vi "InitializeHardware_RT.vi"(1 "PXI card names":string[](array[string])=["DIO:", "6509", "Counter:", "6733_1", "Slow AO:", "6723", "Fast AO:", "6733_1", "6733_2"]) -> (0 "Task cluster":T1={"inbits"=8, "outbits"=38, "Counter"="Counter", "Inbits"="Inbits", "Outbits"="Outbits", "Fast AO"=["FastAO_1", "FastAO_2"], "Errors"={"status"=FALSE, "code"=0, "source"=""}})   [LabVIEW 2018]
uses:
  Target/Tasks_RT.ctl
panel:
  in  "PXI_Trig0 of ao1":tag="/6733_1/PXI_Trig0"
  in  "skipped outbit chans (7)":i32=7
  out "counter trigger":tag="6509/port1/line0"
  in  "Sample rate":dbl=100000.0 format="%#_13g"
  out "counter out":tag="/6733_1/PXI_Trig0"
  in  "Input Cluster":T2={"inbits"=8, "outbits"=38, "Counter"="6733_1", "Digital"="6509", "Fast AO"=["6733_1", "6733_2"], "Task Names"=["Inbits", "Outbits", "Counter", "FastAO_1", "FastAO_2"]}
  # "Tasks and errors"
  # "In (device names)"
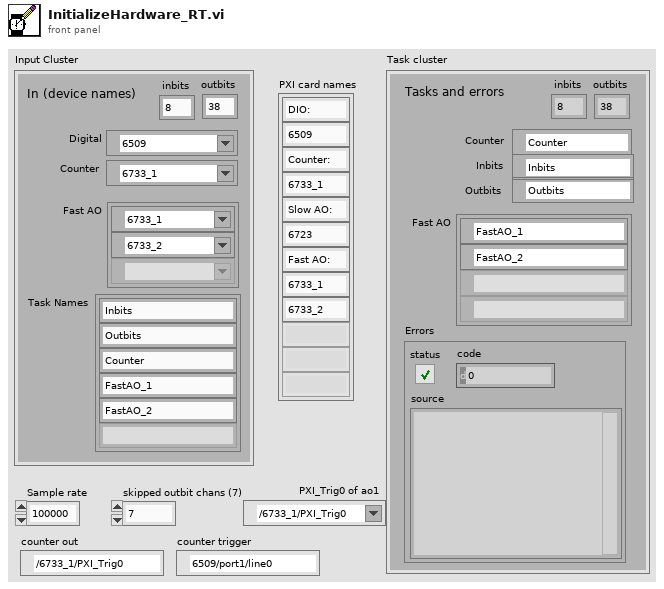
[diagram p1: front panel]
types:
  T1 = typedef "Tasks_RT.ctl" = cluster{"inbits":i32, "outbits":i32, "Counter":refnum<k21>, "Inbits":refnum<k21>, "Outbits":refnum<k21>, "Fast AO":refnum<k21>[], "Errors":errorcluster}
  T2 = cluster{"inbits":i32, "outbits":i32, "Counter":tag, "Digital":tag, "Fast AO":tag[], "Task Names":string[]}
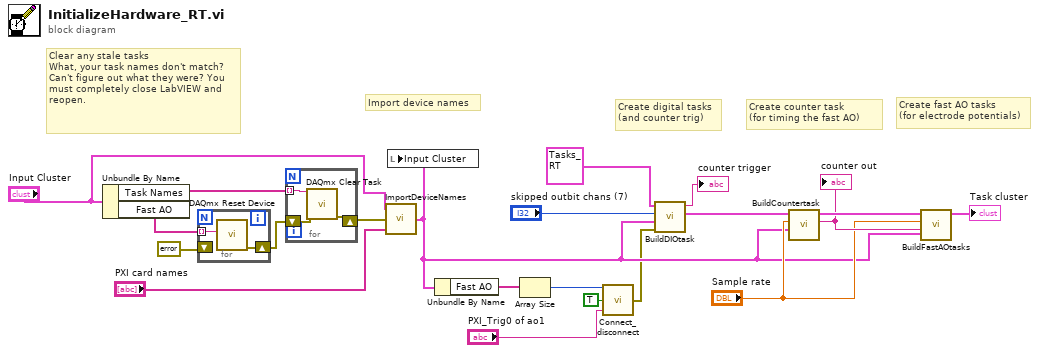
[diagram p0: block diagram]
diagram:
  # "Create fast AO tasks \n(for electrode potentials)"
  # "Create counter task \n(for timing the fast AO)"
  # "Create digital tasks \n(and counter trig)"
  # "Import device names"
  # "Clear any stale tasks\nWhat, your task names don't match? Can't figure out what they were? You must completely close LabVIEW and reopen."
  n1 = Unbundle By Name("Input Cluster") -> ("Task Names"=w18:string[], "Fast AO"=w9:tag[])
  n2 = for {
    tunnel: w9 -> [w23] mode=indexing
    shift-right: [w22] -> w8
    shift-left: errorcluster {"status"=FALSE, "code"=0, "source"=""} ("error out") -> [_]
    n3 = call <vilib>:"DAQmx Reset Device.vi"("device in"=w23) -> ("error out"=w22:errorcluster)  [unwired: 14 in]
  }
  n4 = for {
    tunnel: w18 -> [w26] mode=indexing
    shift-right: [w25] -> w10
    shift-left: w8 -> [w24]
    n5 = call <vilib>:"DAQmx Clear Task.vi"("task in"=w26, "error in"=w24) -> ("error out"=w25:errorcluster)  [unwired: 13 in]
  }
  n6 = call "ImportDeviceNames.vi"("PXI card names"="PXI card names", "Cleared OK?"=w10, "Input Cluster in"="Input Cluster") -> ("Input Cluster out"=w6:T2)
  n7 = local write "Input Cluster"(w6) -> ()
  n8 = Unbundle By Name(w6) -> ("Fast AO"=w3:tag[])
  n9 = Array Size(array=w3) -> (size(s)=w4:i32)
  n10 = call "Connect_disconnect.vi"("PXI_Trig0 of ao1"="PXI_Trig0 of ao1", "Connect?"=TRUE, "Fast AO lines"=w4) -> ("error out"=w5:errorcluster)
  n11 = call "BuildDIOtask.vi"("error in (no error)"=w5, "Input Cluster"=w6, "skipped outbit chans (7)"="skipped outbit chans (7)", "Task cluster in"=T1 {"inbits"=8, "outbits"=38, "Counter"="Counter", "Inbits"="", "Outbits"="", "Fast AO"=["Fast AO_1", "Fast AO_2"], "Errors"={"status"=FALSE, "code"=0, "source"="Outbits"}} ("Task cluster")) -> ("Task cluster out"=w15:T1, "counter trig"=→"counter trigger":tag)  [unwired: 6 in]
  n12 = call "BuildCountertask.vi"("Input Cluster"=w6, "Sample rate"="Sample rate", "Task cluster in"=w15) -> ("CO.Pulse.Term"=w13:tag, "Task cluster out"=w14:T1)  [unwired: 7 in]
  "counter out" <- w13
  n13 = call "BuildFastAOtasks.vi"("Input Cluster"=w6, "counter in"=w13, "Sample rate"="Sample rate", "Task cluster in"=w14) -> ("Task cluster out"=→"Task cluster":T1)  [unwired: 7 in]
